vi "Split.vi"(0 "INPUT STRING":string) -> (1 "temp":dbl, 2 "humid":dbl, 3 "Web":string, 4 "Control1":bool)   [LabVIEW 2022 SP3]
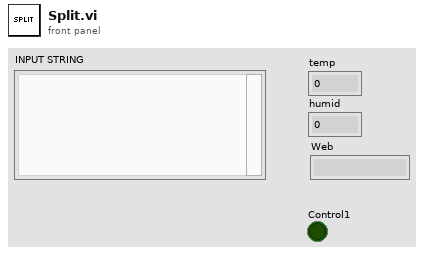
[diagram p1: front panel]
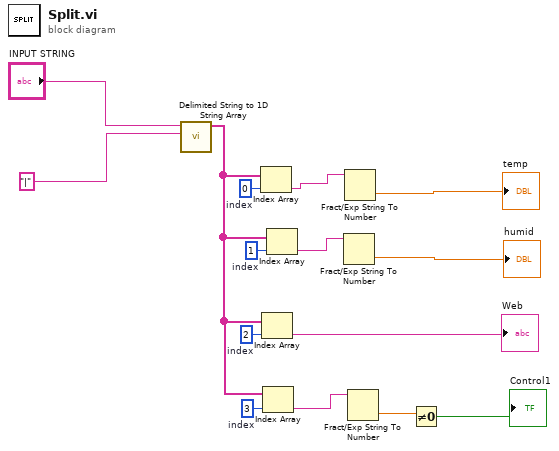
[diagram p0: block diagram]
diagram:
  w5 = 3  # index
  w7 = 2  # index
  w12 = 1  # index
  w13 = 0  # index
  n1 = call <vilib>:"Delimited String to 1D String Array.vi"("delimiter"="|", "delimited string"="INPUT STRING") -> ("string array"=w4:string[])  [unwired: 9 in]
  n2 = Index Array "Index Array"(array=w4, index=w13) -> (element=w11:string)
  n3 = Index Array "Index Array"(array=w4, index=w7) -> (element=→"Web":string)
  n4 = Index Array "Index Array"(array=w4, index=w5) -> (element=w3:string)
  n5 = Index Array "Index Array"(array=w4, index=w12) -> (element=w9:string)
  n6 = Fract/Exp String To Number(string=w9) -> (number=→"humid":dbl)  [unwired: 3 in, 1 out]
  n7 = Fract/Exp String To Number(string=w11) -> (number=→"temp":dbl)  [unwired: 3 in, 1 out]
  n8 = Fract/Exp String To Number(string=w3) -> (number=w2:dbl)  [unwired: 3 in, 1 out]
  n9 = Not Equal To 0?(x=w2) -> (x != 0?=→"Control1":bool)
